vi "SRingStartThreadSD.vi"(0 "releasems":i16=2, 1 "threadp":u32=31, 2 "ringdepth":u32) -> ()   [LabVIEW 2015]
uses:
  DLL/ESLSCDLL.dll
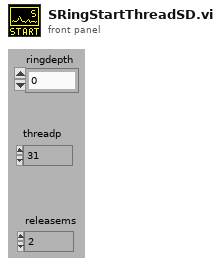
[diagram p1: front panel]
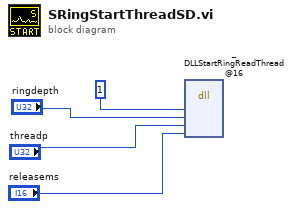
[diagram p0: block diagram]
diagram:
  n1 = dll-call lib="G:/SD/TRANCON/DLL/ESLSCDLL.dll" fn="_DLLStartRingReadThread@16" ("lwlscdll.dll:DLLStartRingReadThread")("drv"=u32 1, "ringdepth"="ringdepth", "threadp"="threadp", "releasems"="releasems") -> ()  [unwired: 8 in, 2 out]
